vi "Sub_SpeedCalc.vi"() -> (6 "a":dbl, 7 "b":dbl)   [LabVIEW 2016]
panel:
  in  "Max":dbl=120.0
  in  "Min":dbl=15.0
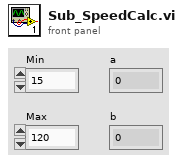
[diagram p1: front panel]
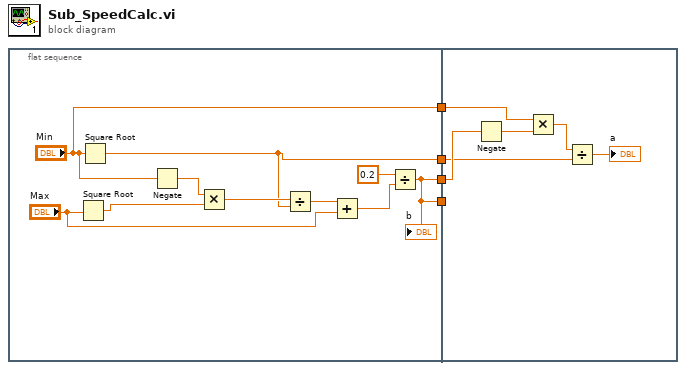
[diagram p0: block diagram]
diagram:
  n1 = flat-sequence {
    tunnel: [w5] -> w4
    tunnel: ["Min"] -> w3
    tunnel: [w6] -> w2
    tunnel: [w5] -> w1
    tunnel: w4 -> [w20]
    tunnel: w3 -> [w18]
    tunnel: w2 -> [w15]
    tunnel: w1 -> [_]
    frame #0 {
      n2 = Square Root(x="Max") -> (sqrt(x)=w12:dbl)
      n3 = Square Root(x="Min") -> (sqrt(x)=w6:dbl)
      n4 = Negate(x="Min") -> (-x=w13:dbl)
      n5 = Multiply(x=w13, y=w12) -> (x*y=w11:dbl)
      n6 = Divide(x=w11, y=w6) -> (x/y=w10:dbl)
      n7 = Add(x=w10, y="Max") -> (x+y=w8:dbl)
      n8 = Divide(x=0.2, y=w8) -> (x/y=w5:dbl)
      "b" <- w5
    }
    frame #1 {
      n9 = Negate(x=w20) -> (-x=w19:dbl)
      n10 = Multiply(x=w18, y=w19) -> (x*y=w17:dbl)
      n11 = Divide(x=w17, y=w15) -> (x/y=→"a":dbl)
    }
  }
